vi "nipkg-setPackageName.vi"(8 "error in (no error)":errorcluster, 9 "VeriStand Version":string, 10 "Package name":string, 11 "Project refs":T1={"LabVIEW Project Path"=path "C:/Users/admin/Desktop/Source/Waveform-Processing-Custom-Device.lvproj", "Project refnum"=refnum, "Build spec refnum"=refnum}) -> (0 "error out":errorcluster, 2 "Updated package name":string, 3 "Project refs out":T1={"LabVIEW Project Path"=path "C:/Users/admin/Desktop/Source/Waveform-Processing-Custom-Device.lvproj", "Project refnum"=refnum, "Build spec refnum"=refnum})   [LabVIEW 2014, in "nipkg-build-system.lvlib"]
uses:
  nipkg-build-system.lvlib
  lv-build-system/lv-build-library.lvlib
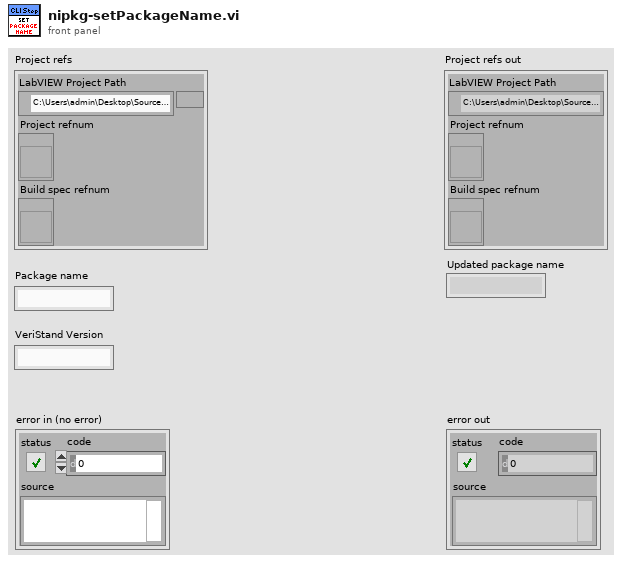
[diagram p1: front panel]
types:
  T1 = cluster{"LabVIEW Project Path":path, "Project refnum":refnum<vi>, "Build spec refnum":refnum<vi>}
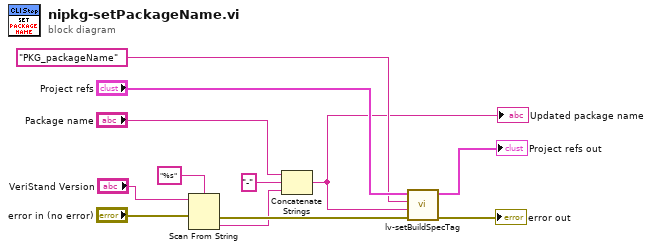
[diagram p0: block diagram]
diagram:
  n1 = Scan From String(format string="%s", input string="VeriStand Version", error in="error in (no error)") -> (error out=w6:errorcluster, output 1=w2:string)  [unwired: 2 in, 2 out]
  n2 = Concatenate Strings("Package name", "-" ("string"), w2) -> (w3:string)
  "Updated package name" <- w3
  n3 = call "lv-setBuildSpecTag.vi"("error in (no error)"=w6, "Tag value"=w3, "Tag name"="PKG_packageName", "Project refs"="Project refs") -> ("error out"=→"error out":errorcluster, "Project refs out"=→"Project refs out":T1)  [unwired: 6 in]
